vi "ExternalSetParam.vi"(0 "reference in":refnum<class "VINode.lvclass">, 1 "setParameter":T2, 2 "string":string, 3 "Position":T1 {"y" format="%.2f"; "x" format="%.2f"}, 5 "error in (no error)":errorcluster, 7 "ClassPath":path) -> (14 "reference out":refnum<class "VINode.lvclass">, 19 "error out":errorcluster)   [LabVIEW 2016, in "VINode.lvclass"]
doc: "Sets parameter externaly.\nPossible to set Name,Attrib,Methods and Position"
uses:
  <resource>/Framework/Providers/Open_GDS/UML/VINode_class/VINode.lvclass
  C:/Program Files (x86)/National Instruments/LabVIEW 2016/resource/Framework/Providers/Open_GDS/UML/RectangularNode_class/RectangularNode.lvclass
  <resource>/Framework/Providers/Open_GDS/UML/VINode_class/ExternalSetTypes.ctl
  <resource>/Framework/Providers/Open_GDS/UML/General/Point/Point Point2D.ctl
  <resource>/Framework/Providers/Open_GDS/UML/MultiLineString_class/MultiLineString.lvclass
  <resource>/Framework/Providers/Open_GDS/UML/RectangularNode_class/RectangularNode.lvclass
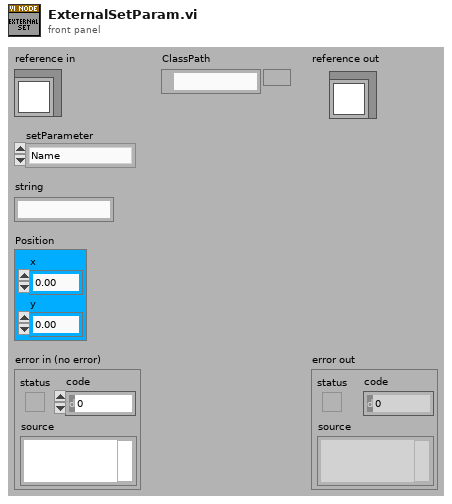
[diagram p1: front panel]
types:
  T1 = typedef "Point Point2D.ctl" = cluster{"x":dbl, "y":dbl}
  T2 = typedef "VINode.lvclass/ExternalSetTypes.ctl" = enum16{"Name", "ClassPath", "Position", "Description"}
  T3 = typedef "VINode.lvclass/ObjectAttributes.ctl" = cluster{"midHeight":dbl, "botHeight":dbl, "Name":refnum<class "MultiLineString.lvclass">, "DEFAULT_COMPARTMENT_HEIGHT":i32, "DEFAULT_WIDTH":i32, "DEFAULT_HEIGHT":i32, "VIPath":path, "Description":refnum<class "MultiLineString.lvclass">, "ShowDescription":bool}
  T4 = typedef "RectangularNode.lvclass/ObjectAttributes.ctl" = cluster{"bounds":T5}
  T5 = typedef "Rectangle Rectangle2D.ctl" = cluster{"x":dbl, "y":dbl, "width":dbl, "height":dbl}
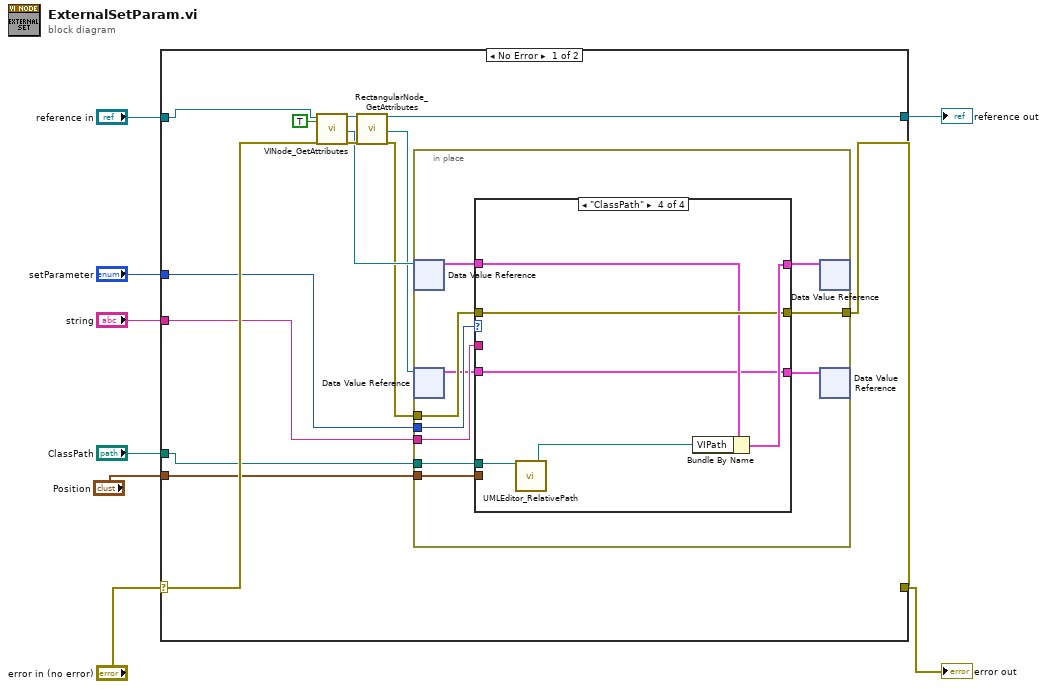
[diagram p0: block diagram]
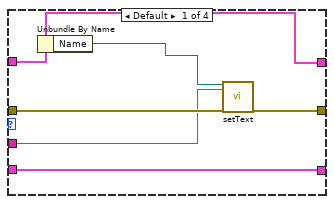
[diagram p2: hidden frame]
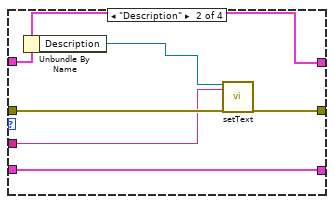
[diagram p3: hidden frame]
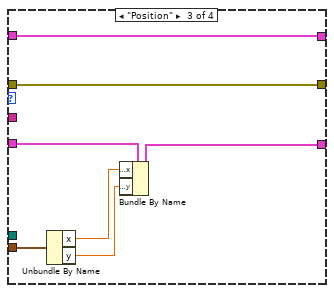
[diagram p4: hidden frame]
diagram:
  n1 = case shown="No Error" "error in (no error)" {
    selector: "error in (no error)" -> [w19 w58]
    tunnel: "reference in" -> [w22 w59]
    tunnel: [w21 w58] -> w6
    tunnel: [w20 w59] -> w5
    tunnel: "setParameter" -> [w13 _]
    tunnel: "string" -> [w11 _]
    tunnel: "ClassPath" -> [w10 _]
    tunnel: "Position" -> [w9 _]
    frame No Error {
      n2 = call <resource>:"VINode_GetAttributes.vi"("reference in"=w22, "OnlyGetDvrReference(False)"=TRUE, "error in (no error)"=w19) -> ("reference out"=w17:refnum<class "VINode.lvclass">, "DataRef"=w15:refnum<data-value>, "error out"=w16:errorcluster)  [unwired: 13 in, 1 out]
      n3 = call <resource>:"RectangularNode_GetAttributes.vi"("reference in"=w17, "error in (no error)"=w16) -> ("reference out"=w20:refnum<class "VINode.lvclass">, "DataRef"=w14:refnum<data-value>, "error out"=w12:errorcluster)  [unwired: 14 in, 1 out]
      n4 = in-place {
        in-place-border: w13 -> [w32]
        in-place-border: w12 -> [w31]
        in-place-border: w11 -> [w30]
        in-place-border: w10 -> [w29]
        in-place-border: [w26] -> w21
        in-place-border: w9 -> [w23]
        n5 = in-place-dvr #1(w15) -> (w28:T3)  [unwired: 1 out]
        n6 = in-place-dvr #2(w14) -> (w27:T4)  [unwired: 1 out]
        n7 = case shown="\"ClassPath\"" w32 {
          tunnel: [w34 w40 w46 w57] -> w25
          tunnel: w31 -> [w38 w44 w49 w56]
          tunnel: [w37 w43 w49 w56] -> w26
          tunnel: w30 -> [w36 w42 _ _]
          tunnel: w29 -> [_ _ _ w54]
          tunnel: w28 -> [w34 w40 w46 w53]
          tunnel: w27 -> [w33 w39 w48 w52]
          tunnel: [w33 w39 w47 w52] -> w24
          tunnel: w23 -> [_ _ w45 _]
          frame Default {
            n8 = Unbundle By Name(w34) -> ("Name"=w35:refnum<class "MultiLineString.lvclass">)
            n9 = call-dynamic "setText.vi"("reference"=w35, "text"=w36, "error in (no error)"=w38) -> ("error out"=w37:errorcluster)  [unwired: 16 out]
          }
          frame "Description" {
            n10 = Unbundle By Name(w40) -> ("Description"=w41:refnum<class "MultiLineString.lvclass">)
            n11 = call-dynamic "setText.vi"("reference"=w41, "text"=w42, "error in (no error)"=w44) -> ("error out"=w43:errorcluster)  [unwired: 16 out]
          }
          frame "Position" {
            n12 = Unbundle By Name(w45) -> ("x"=w51:dbl, "y"=w50:dbl)
            n13 = Bundle By Name(cluster=w48, "bounds.x"=w51, "bounds.y"=w50) -> (w47:T4)
          }
          frame "ClassPath" {
            n14 = call <resource>:"UMLEditor_RelativePath.vi"("Path In"=w54) -> ("ConvertToRelativePath(If possible)"=w55:path)  [unwired: 1 in, 17 out]
            n15 = Bundle By Name(cluster=w53, "VIPath"=w55) -> (w57:T3)
          }
        }
        n16 = in-place-dvr #1(w25) -> ()  [unwired: 2 out]
        n17 = in-place-dvr #2(w24) -> ()  [unwired: 2 out]
      }
    }
    frame Error {
    }
  }
  "reference out" <- w5
  "error out" <- w6
